vi "FA_AgentConfig_GetRevision.vi"(2 "Dev":bool, 3 "Current VI Path":path, 5 "Error In":errorcluster) -> (14 "Revision String":string, 15 "MajorRev":i32, 16 "MinorRev":i32, 17 "IterationNum":i32, 18 "BuildNum":i32, 19 "Error Out":errorcluster)   [LabVIEW 2014, in "FA_AgentConfig.lvlib"]
doc: "Returns the current build revision number for FlockAgent."
uses:
  FA_AgentConfig.lvlib
  <vilib>/Utility/config.llb/Read Key (I32).vi
  <vilib>/Utility/config.llb/NI_LVConfig.lvlib
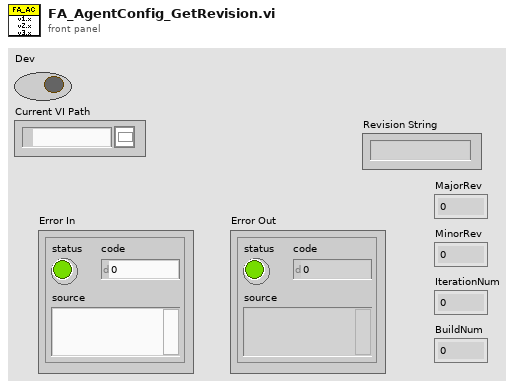
[diagram p1: front panel]
types:
  T1 = typedef "FA_AgentConfig.lvlib/FA_AgentConfig_Refnum.ctl" = cluster{"INI  Refnum":T2}
  T2 = typedef "NI_LVConfig.lvlib/Config Data RefNum.ctl" = refnum<k1>
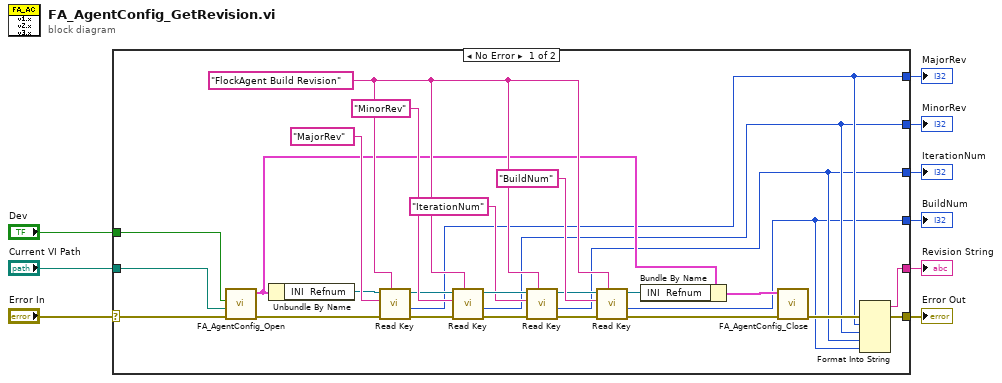
[diagram p0: block diagram]
diagram:
  n1 = case shown="No Error" "Error In" {
    selector: "Error In" -> [w22 w37]
    tunnel: [w15 w37] -> w8
    tunnel: "Dev" -> [w24 _]
    tunnel: "Current VI Path" -> [w23 _]
    tunnel: [w12 _] -> w5
    tunnel: [w13 _] -> w4
    tunnel: [w11 _] -> w3
    tunnel: [w14 _] -> w2
    tunnel: [w10 _] -> w1
    frame No Error {
      w29 = "FlockAgent Build Revision"
      n2 = call "FA_AgentConfig_Open.vi"("Error In"=w22, "Current VI Path"=w23, "Dev"=w24) -> ("Error Out"=w21:errorcluster, "INI File Path"=w19:T1)  [unwired: 7 in]
      n3 = Unbundle By Name(w19) -> ("INI  Refnum"=w25:T2)
      n4 = call-poly <vilib>:"Read Key.vi"("section"=w29, "error in (no error)"=w21, "key"="MajorRev", "refnum"=w25) -> ("error out"=w34:errorcluster, "value"=w14:i32, "refnum out"=w33:T2)  [unwired: 4 in, 1 out]
      n5 = call-poly <vilib>:"Read Key.vi"("section"=w29, "error in (no error)"=w34, "key"="MinorRev", "refnum"=w33) -> ("error out"=w31:errorcluster, "value"=w13:i32, "refnum out"=w30:T2)  [unwired: 4 in, 1 out]
      n6 = call-poly <vilib>:"Read Key.vi"("section"=w29, "error in (no error)"=w31, "key"="IterationNum", "refnum"=w30) -> ("error out"=w27:errorcluster, "value"=w12:i32, "refnum out"=w26:T2)  [unwired: 4 in, 1 out]
      n7 = call-poly <vilib>:"Read Key.vi"("section"=w29, "error in (no error)"=w27, "key"="BuildNum", "refnum"=w26) -> ("error out"=w20:errorcluster, "value"=w11:i32, "refnum out"=w18:T2)  [unwired: 4 in, 1 out]
      n8 = Bundle By Name(cluster=w19, "INI  Refnum"=w18) -> (w17:T1)
      n9 = call "FA_AgentConfig_Close.vi"("Error In"=w20, "FA_AgentConfig_Refnum 2"=w17) -> ("Error Out"=w16:errorcluster)  [unwired: 9 in]
      n10 = Format Into String(error in=w16, w14, w13, w12, w11) -> (resulting string=w10:string, error out=w15:errorcluster)  [unwired: 2 in]
    }
    frame Error {
    }
  }
  "Error Out" <- w8
  "IterationNum" <- w5
  "MinorRev" <- w4
  "BuildNum" <- w3
  "MajorRev" <- w2
  "Revision String" <- w1
